vi "Configuration SubVI.vi"(8 "error in (no error)":errorcluster, 11 "Simulation in":refnum<class "Simulation.lvclass">) -> (0 "error out":errorcluster, 3 "Simulation out":refnum<class "Simulation.lvclass">)   [LabVIEW 2020, in "Generic I2C.lvlib" / "Simulation.lvclass"]
uses:
  Simulation.lvclass
  C:/Users/kaiser.asan/OneDrive - SolitonTechnologies/LabVIEW/29.SDLC - I2C Driver/I2C Module/I2C Controller Module/Class/Devices/Child/Generic I2C/Parent/Generic I2C.lvclass
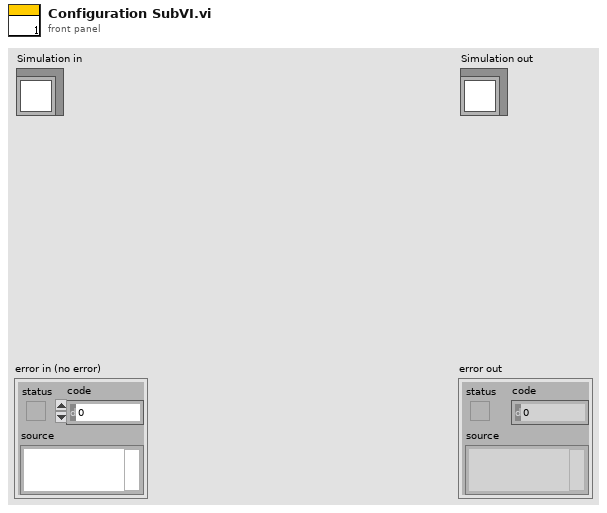
[diagram p1: front panel]
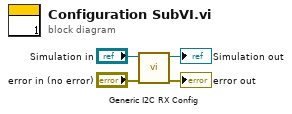
[diagram p0: block diagram]
diagram:
  n1 = call "Generic I2C RX Config.vi"("error in (no error)"="error in (no error)", "Generic I2C.lvclass In"="Simulation in") -> ("error out"=→"error out":errorcluster, "Generic I2C.lvclass Out"=→"Simulation out":refnum<class "Simulation.lvclass">)  [unwired: 8 in]
